vi "fgt set valve position.vi"(6 "wait (true)":bool=TRUE, 8 "error in (no error)":errorcluster, 9 "direction (shortest)":T1, 10 "position":i32, 11 "valveIndex":u32) -> (0 "error out":errorcluster)   [LabVIEW 2020, in "fgt_SDK.lvlib"]
doc: "Switch valve to the requested position. If Wait is true, block until the valve arrives at the position.\nIf the valve is an M-Switch, the direction input specifies in which direction it should turn."
uses:
  fgt_SDK.lvlib
  TypeDefs/fgt_SWITCH_DIRECTION.ctl
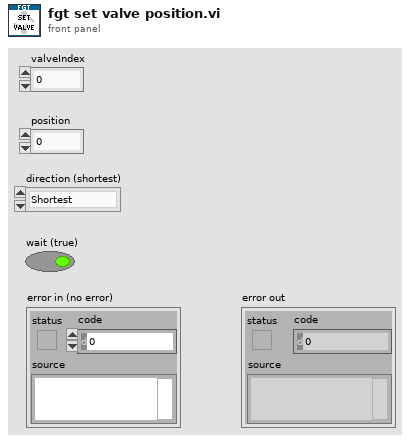
[diagram p1: front panel]
types:
  T1 = typedef "fgt_SDK.lvlib/fgt_SWITCH_DIRECTION.ctl" = enum16{"Shortest", "Anticlockwise", "Clockwise"}
  T2 = typedef "fgt_SDK.lvlib/fgt_STATUS_INFO.ctl" = cluster{"InstrType":T3, "instrSN":u16, "errorCode":u8, "infoCode":u8, "detail":string}
  T3 = typedef "fgt_SDK.lvlib/fgt_INSTRUMENT_TYPE.ctl" = enum32{"None", "MFCS", "MFCS_EZ", "FRP", "LineUP", "IPS"}
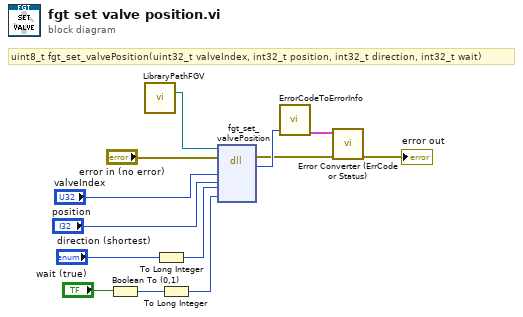
[diagram p0: block diagram]
diagram:
  # "uint8_t fgt_set_valvePosition(uint32_t valveIndex, int32_t position, int32_t direction, int32_t wait)"
  n1 = Boolean To (0,1)(Boolean="wait (true)") -> (0, 1=w9:i16)
  n2 = call "LibraryPathFGV.vi"() -> ("Path Out"=w1:path)  [unwired: 14 in, 1 out]
  n3 = To Long Integer(number="direction (shortest)") -> (32bit integer=w2:i32)
  n4 = To Long Integer(number=w9) -> (32bit integer=w8:i32)
  n5 = dll-call lib="C:/Workspace/fgt-SDK/LabVIEW/dlls/fgt_SDK_*.*" fn="fgt_set_valvePosition"(path in=w1, error in="error in (no error)", "valveIndex"="valveIndex", "position"="position", "direction"=w2, "wait"=w8) -> (error out=w5:errorcluster, "return type"=w7:u8)  [unwired: 5 in, 1 out]
  n6 = call "ErrorCodeToErrorInfo.vi"("return type"=w7) -> ("StatusInfo"=w6:T2)  [unwired: 10 in]
  n7 = call "Error Converter (ErrCode or Status).vi"("error in (no error)"=w5, "StatusInfo"=w6) -> ("error out"=→"error out":errorcluster)  [unwired: 9 in]
